vi "createTestCaseXML.vi"(7 "TestTestResult.Ant":refnum<class "_TextTestResult.JUnitXML.lvclass">, 8 "error in (no error)":errorcluster, 9 "execution time (sec)":dbl, 10 "resultStatus":T1, 11 "Test Out":refnum<class>) -> (0 "error out":errorcluster, 5 "TestTestResult.Ant Out":refnum<class "_TextTestResult.JUnitXML.lvclass">)   [LabVIEW 2011, in "_TextTestResult.JUnitXML.lvclass"]
uses:
  _TextTestResult.JUnitXML.lvclass
  <vilib>/addons/_JKI Toolkits/VI Tester/TestResult.llb/resultStatus--enum.ctl
  JUnitXML.ResultXML--TestCaseAttributes.ctl
  <vilib>/addons/_JKI Toolkits/VI Tester/TestSuite.llb/TestSuite.lvclass
  JUnitXML.ResultXML.ctl
  JUnitXML.ResultXML--TestSuiteAttributes.ctl
  _TextTestResult.JUnitXML.lvclass/_TextTestResult.JUnitXML.ctl
  <vilib>/addons/_JKI Toolkits/VI Tester/TestResult.llb/TestResult.lvclass
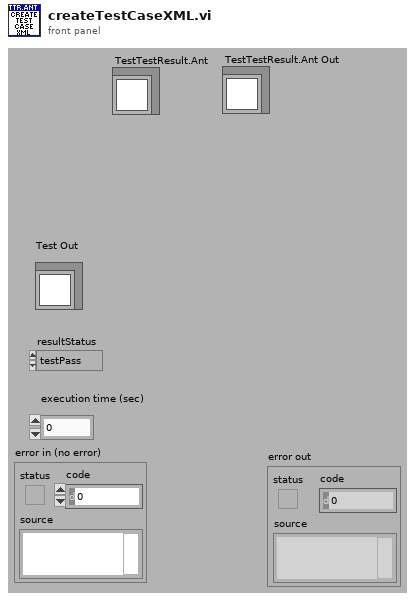
[diagram p1: front panel]
types:
  T1 = typedef "TestResult.lvclass/resultStatus--enum.ctl" = enum16{"testPass", "testFailure", "testError", "testSkipped"}
  T2 = typedef "_TextTestResult.JUnitXML.lvclass/JUnitXML.ResultXML--TestCaseAttributes.ctl" = cluster{"classname":string, "name":string, "time":dbl}
  T3 = cluster{"#attributes":T2, "failure":cluster{"#attributes":cluster{"message":string, "type":string}, "failure":string}}
  T4 = typedef "TestResult.lvclass/failure.ctl" = cluster{"test":refnum<class>, "error":errorcluster}
  T5 = cluster{"#attributes":T2, "error":cluster{"#attributes":cluster{"message":string, "type":string}, "error":string}}
  T6 = typedef "TestResult.lvclass/errors.ctl" = T7[]
  T7 = typedef "TestResult.lvclass/error.ctl" = cluster{"test":refnum<class>, "error":errorcluster}
  T8 = cluster{"#attributes":T2, "skipped":cluster{"skipped":string}}
  T9 = typedef "TestResult.lvclass/skipped.ctl" = T10[]
  T10 = typedef "TestResult.lvclass/skip.ctl" = cluster{"test":refnum<class>, "error":errorcluster}
  T11 = typedef "_TextTestResult.JUnitXML.lvclass/JUnitXML.ResultXML.ctl" = cluster{"#attributes":T12, "testsuite":cluster{"#attributes":T12, "testcase":T2[]}[]}
  T12 = typedef "_TextTestResult.JUnitXML.lvclass/JUnitXML.ResultXML--TestSuiteAttributes.ctl" = cluster{"name":string}
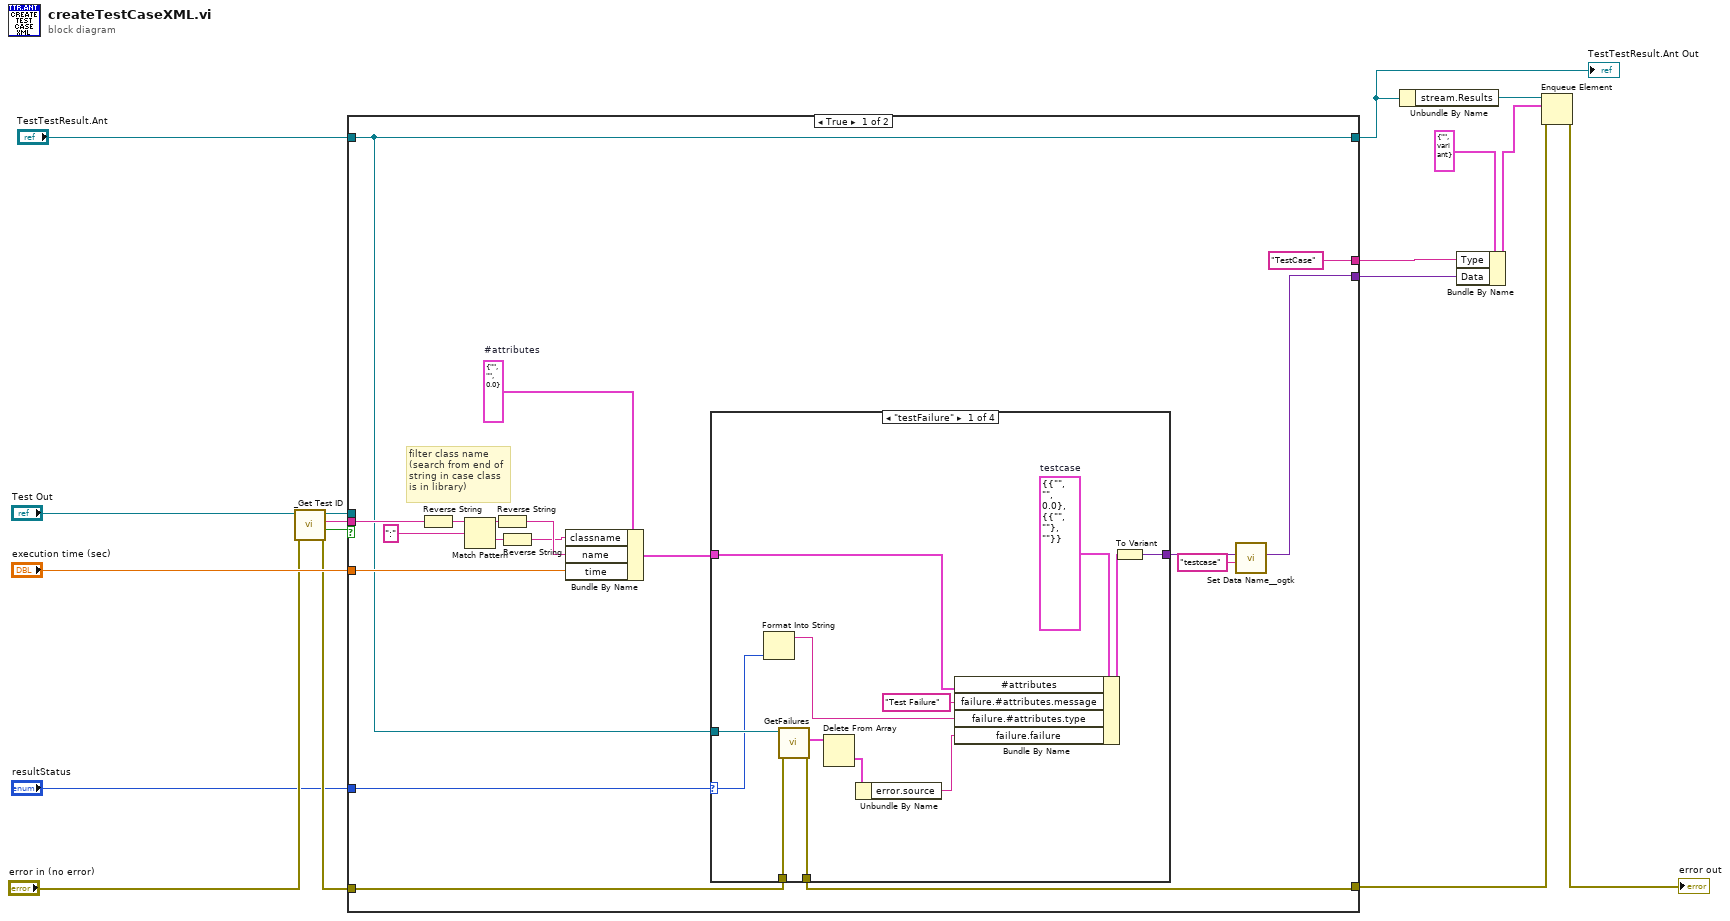
[diagram p0: block diagram]
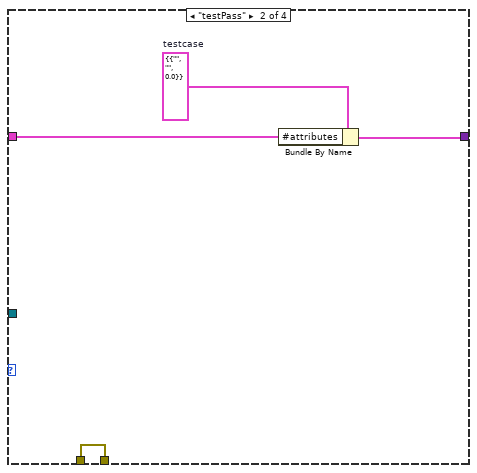
[diagram p2: hidden frame]
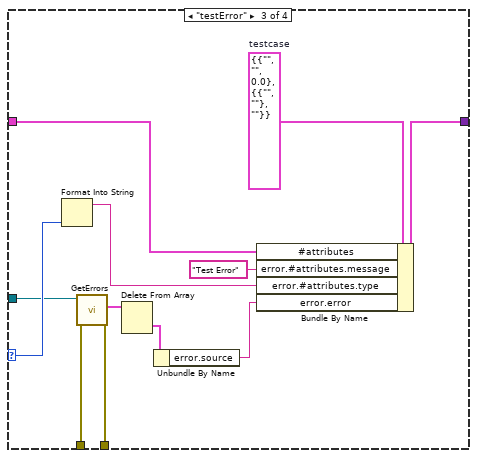
[diagram p3: hidden frame]
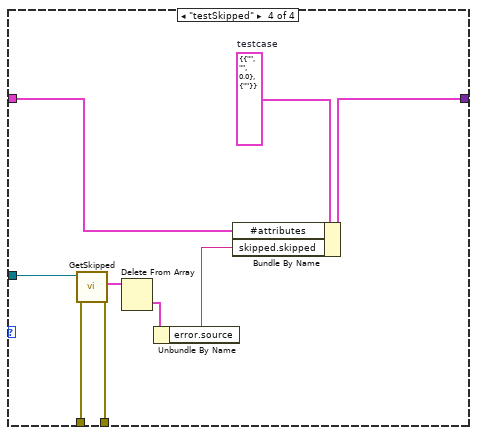
[diagram p4: hidden frame]
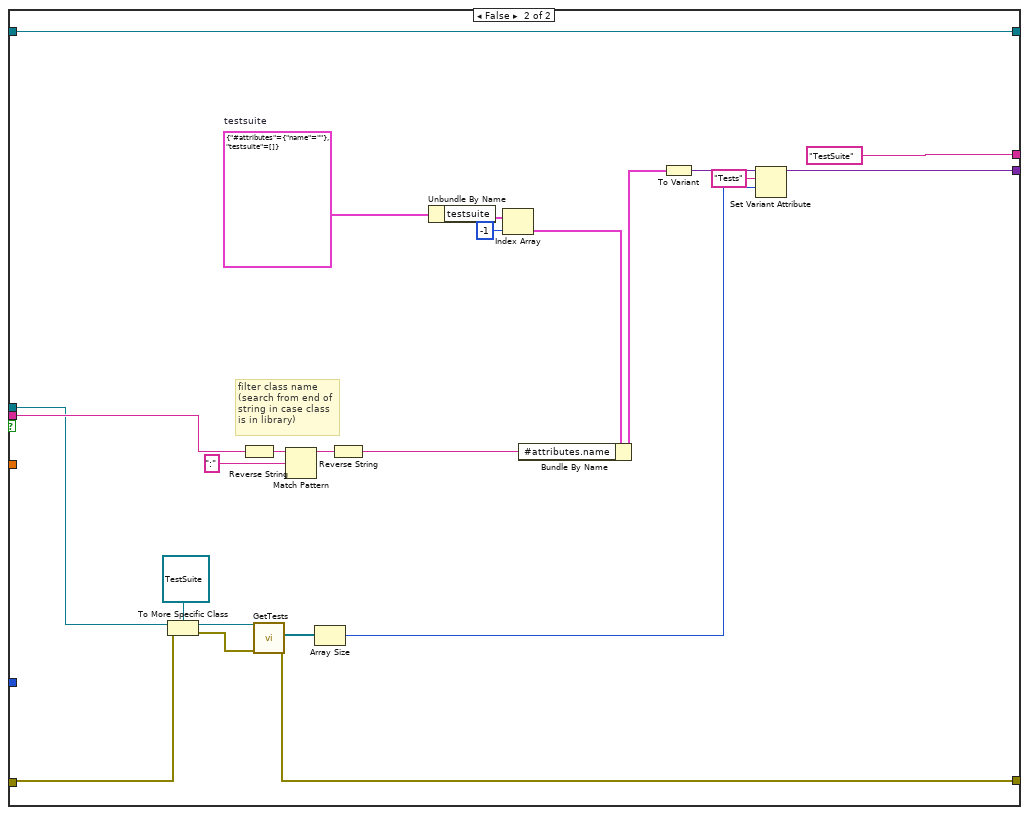
[diagram p5: hidden frame]
diagram:
  n1 = call "_Get Test ID.vi"("error in"="error in (no error)", "Test In"="Test Out") -> ("error out"=w4:errorcluster, "IsTestCase"=w12:bool, "id"=w16:string, "Test Out"=w14:refnum<class>)  [unwired: 5 in, 1 out]
  n2 = case shown="True" w12 {
    tunnel: "execution time (sec)" -> [w35 _]
    tunnel: w16 -> [w31 w93]
    tunnel: w14 -> [_ w84]
    tunnel: w4 -> [w25 w79]
    tunnel: [w24 w78] -> w6
    tunnel: ["TestCase" "TestSuite"] -> w9
    tunnel: [w20 w76] -> w8
    tunnel: [w23 w77] -> w2
    tunnel: "TestTestResult.Ant" -> [w23 w77]
    tunnel: "resultStatus" -> [w26 _]
    frame True {
      w22 = T2 {"classname"="", "name"="", "time"=0.0}  # #attributes
      # "filter class name\n(search from end of string in case class is in library)"
      n3 = Reverse String(1:w31) -> (0:w33:string)
      n4 = Match Pattern(string=w33, regular expression=":") -> (before substring=w32:string, after substring=w29:string)  [unwired: 1 in, 2 out]
      n5 = Reverse String(1:w32) -> (0:w30:string)
      n6 = Reverse String(1:w29) -> (0:w28:string)
      n7 = Bundle By Name(cluster=w22, "classname"=w28, "name"=w30, "time"=w35) -> (w21:T2)
      n8 = case shown="\"testFailure\"" w26 {
        selector: w26 -> [w42 _ w62 _]
        tunnel: w21 -> [w37 w50 w53 w65]
        tunnel: [w36 w49 w64 w73] -> w19
        tunnel: w23 -> [w47 _ w58 w71]
        tunnel: w25 -> [w46 w52 w56 w70]
        tunnel: [w45 w52 w55 w69] -> w24
        frame "testFailure" {
          w38 = T3 {"#attributes"={"classname"="", "name"="", "time"=0.0}, "failure"={"#attributes"={"message"="", "type"=""}, "failure"=""}}  # testcase
          n9 = Format Into String(w42) -> (resulting string=w41:string)  [unwired: 3 in, 1 out]
          n10 = call-dynamic "GetFailures.vi"("error in (no error)"=w46, "TestResult in"=w47) -> ("error out"=w45:errorcluster, "failures"=w44:T4[])  [unwired: 7 in, 1 out]
          n11 = Delete From Array(array=w44) -> (deleted portion=w43:T4)  [unwired: 2 in, 1 out]
          n12 = Unbundle By Name(w43) -> ("error.source"=w40:string)
          n13 = Bundle By Name(cluster=w38, "#attributes"=w37, "failure.#attributes.message"="Test Failure", "failure.#attributes.type"=w41, "failure.failure"=w40) -> (w48:T3)
          n14 = To Variant(anything=w48) -> (Variant=w36:variant)
        }
        frame "testPass" {
          w51 = cluster{"#attributes":T2} {"#attributes"={"classname"="", "name"="", "time"=0.0}}  # testcase
          n15 = Bundle By Name(cluster=w51, "#attributes"=w50) -> (w49:cluster{"#attributes":T2})
        }
        frame "testError" {
          w54 = T5 {"#attributes"={"classname"="", "name"="", "time"=0.0}, "error"={"#attributes"={"message"="", "type"=""}, "error"=""}}  # testcase
          n16 = Format Into String(w62) -> (resulting string=w61:string)  [unwired: 3 in, 1 out]
          n17 = call-dynamic "GetErrors.vi"("error in (no error)"=w56, "TestResult in"=w58) -> ("error out"=w55:errorcluster, "Errors"=w57:T6)  [unwired: 7 in, 1 out]
          n18 = Delete From Array(array=w57) -> (deleted portion=w63:T7)  [unwired: 2 in, 1 out]
          n19 = Unbundle By Name(w63) -> ("error.source"=w60:string)
          n20 = Bundle By Name(cluster=w54, "#attributes"=w53, "error.#attributes.message"="Test Error" ("failure.#attributes.message"), "error.#attributes.type"=w61, "error.error"=w60) -> (w64:T5)
        }
        frame "testSkipped" {
          w66 = T8 {"#attributes"={"classname"="", "name"="", "time"=0.0}, "skipped"={"skipped"=""}}  # testcase
          n21 = call-dynamic "GetSkipped.vi"("error in (no error)"=w70, "TestResult in"=w71) -> ("error out"=w69:errorcluster, "Skipped"=w68:T9)  [unwired: 7 in, 1 out]
          n22 = Delete From Array(array=w68) -> (deleted portion=w72:T10)  [unwired: 2 in, 1 out]
          n23 = Unbundle By Name(w72) -> ("error.source"=w67:string)
          n24 = Bundle By Name(cluster=w66, "#attributes"=w65, "skipped.skipped"=w67) -> (w73:T8)
        }
      }
      n25 = call <userlib>:"Set Data Name__ogtk.vi"("Data Name"="testcase", "Data"=w19) -> ("Renamed Data"=w20:variant)  [unwired: 8 in, 1 out]
    }
    frame False {
      w91 = T11 {"#attributes"={"name"=""}, "testsuite"=[]}  # testsuite
      # "filter class name\n(search from end of string in case class is in library)"
      n26 = To More Specific Class(target class=refnum<class "TestSuite.lvclass"> refnum ("TestSuite in"), reference=w84, error in=w79) -> (specific class reference=w80:refnum<class "TestSuite.lvclass">, error out=w81:errorcluster)
      n27 = Reverse String(1:w93) -> (0:w95:string)
      n28 = call-dynamic "GetTests.vi"("error in (no error)"=w81, "TestSuite in"=w80) -> ("error out"=w78:errorcluster, "tests"=w83:refnum<class>[])  [unwired: 7 in, 1 out]
      n29 = Match Pattern(string=w95, regular expression=":") -> (before substring=w94:string)  [unwired: 1 in, 3 out]
      n30 = Array Size(array=w83) -> (size(s)=w74:i32)
      n31 = Reverse String(1:w94) -> (0:w92:string)
      n32 = Unbundle By Name(w91) -> ("testsuite"=w90:cluster{"#attributes":T12, "testcase":T2[]}[])
      n33 = Index Array(array=w90, index=-1) -> (element=w88:cluster{"#attributes":T12, "testcase":T2[]})
      n34 = Bundle By Name(cluster=w88, "#attributes.name"=w92) -> (w86:cluster{"#attributes":T12, "testcase":T2[]})
      n35 = To Variant(anything=w86) -> (Variant=w85:variant)
      n36 = Set Variant Attribute(Variant=w85, name="Tests", value=w74) -> (Variant out=w76:variant)  [unwired: 1 in, 2 out]
    }
  }
  "TestTestResult.Ant Out" <- w2
  n37 = Unbundle By Name(w2) -> ("stream.Results"=w5:refnum<queue>)
  n38 = Bundle By Name(cluster=cluster{"Type":string, "Data":variant} {"Type"="", "Data"=variant} ("element"), "Type"=w9, "Data"=w8) -> (w10:cluster{"Type":string, "Data":variant})
  n39 = Enqueue Element(queue=w5, element=w10, error in (no error)=w6) -> (error out=→"error out":errorcluster)  [unwired: 1 in, 2 out]
